vi "RTEH Error Processor.vi"(4 "Valid Default":bool, 6 "Default Action":T2, 8 "Error to Check":errorcluster, 9 "Detect Any Warnings":bool, 10 "Iteration":i32, 11 "Error Handling Info":T2[](array[typedef])) -> (0 "error out":errorcluster, 1 "Loop?":bool, 2 "Classification":string, 5 "Internal Status":cluster{"Status":T1, "Error Code":i32})   [LabVIEW 2024]
doc: "This SubVI exists so that changes made to the underlying error handling code will propagate to existing instances of the Express VI."
uses:
  Controls/RTEH/RTEH Error Options.ctl
  Controls/RTEH/RTEH Shared Error Options.ctl
  Controls/RTEH/RTEH Status Type.ctl
  Controls/Shared/SEH Error Notification Command.ctl
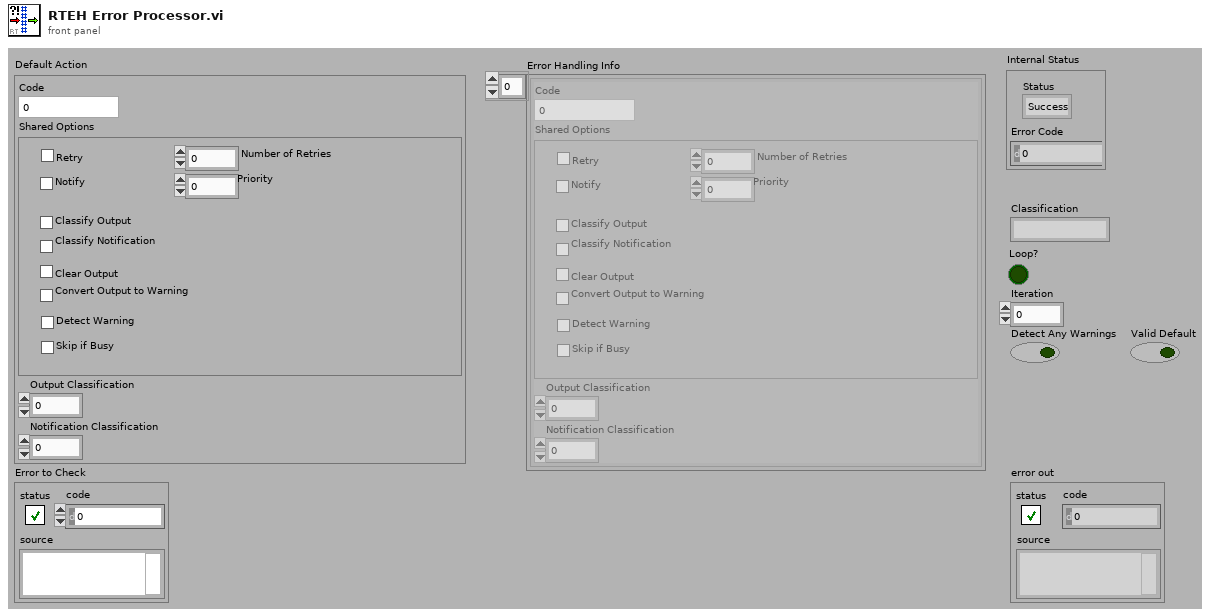
[diagram p1: front panel]
types:
  T1 = typedef "RTEH Status Type.ctl" = enum16{"Success", "Error", "Warning", "Skipped Notification"}
  T2 = typedef "RTEH Error Options.ctl" = cluster{"Code":i32, "Shared Options":T3, "Output Classification":u32, "Notification Classification":u32}
  T3 = typedef "RTEH Shared Error Options.ctl" = cluster{"Number of Retries":i32, "Retry":bool, "Classify Output":bool, "Classify Notification":bool, "Convert Output to Warning":bool, "Clear Output":bool, "Notify":bool, "Priority":i32, "Detect Warning":bool, "Skip if Busy":bool}
  T4 = typedef "SEH Error Notification Command.ctl" = enum16{"Init", "Send Error", "Check Error", "Invalid Command"}
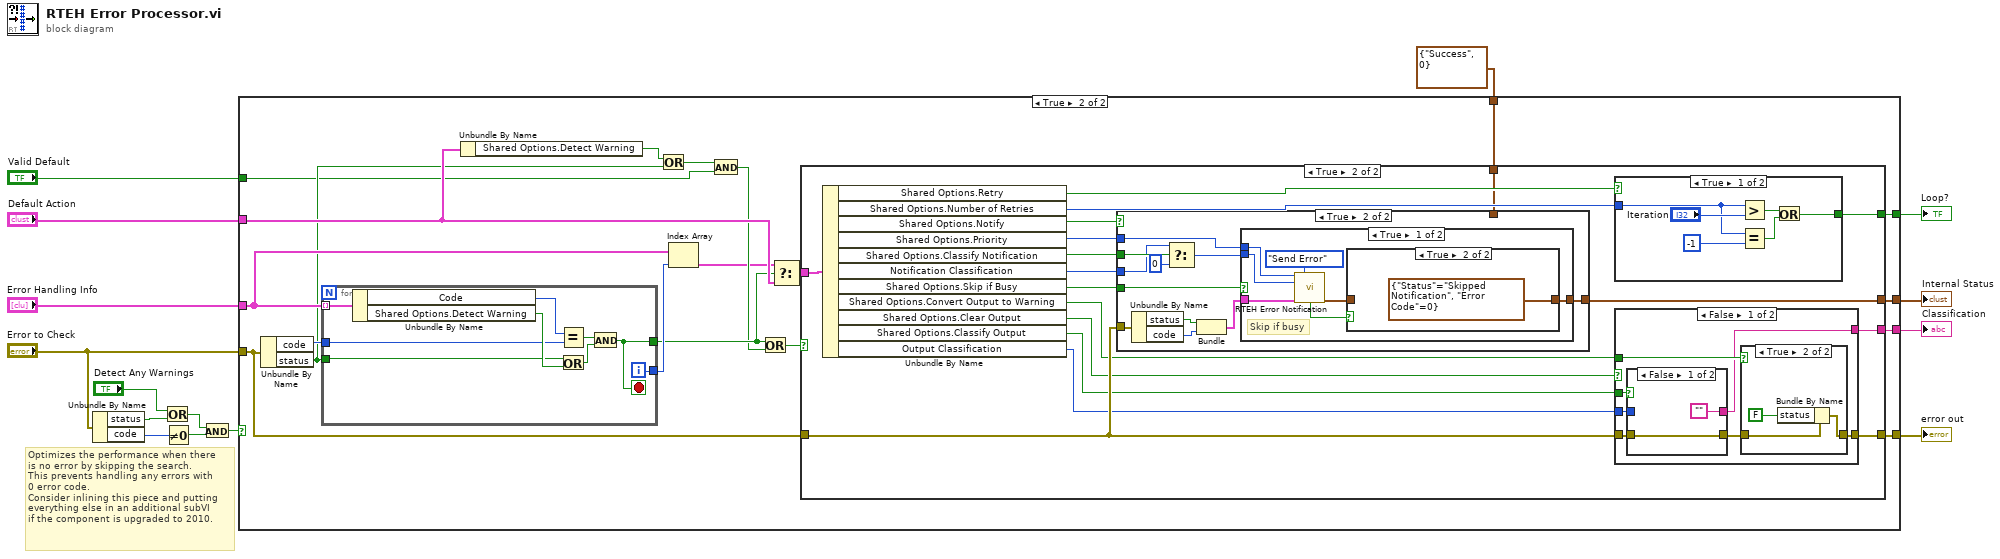
[diagram p0: block diagram]
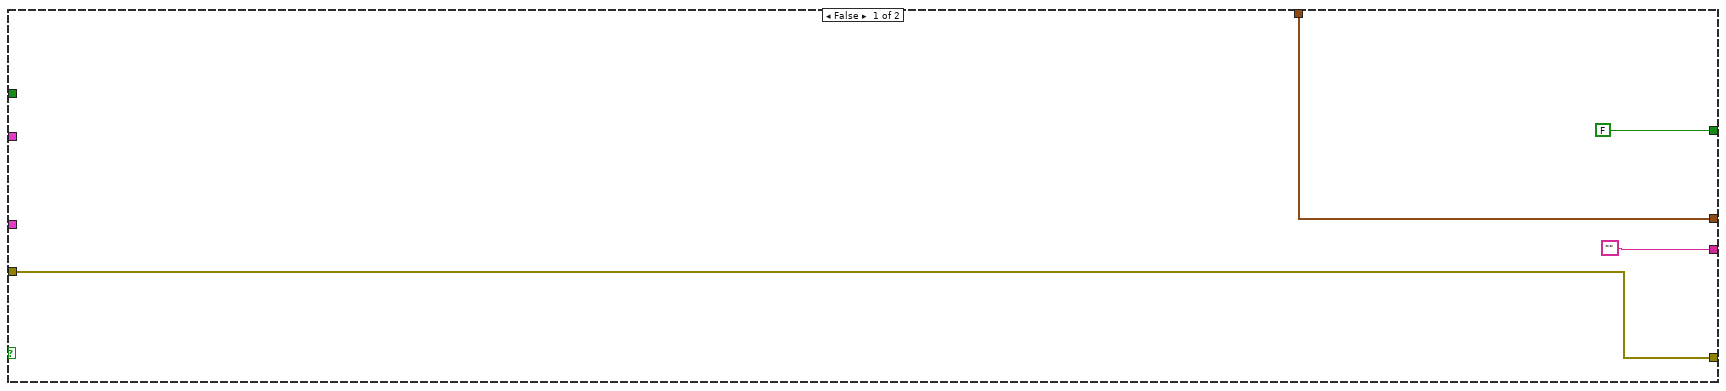
[diagram p2: hidden frame]
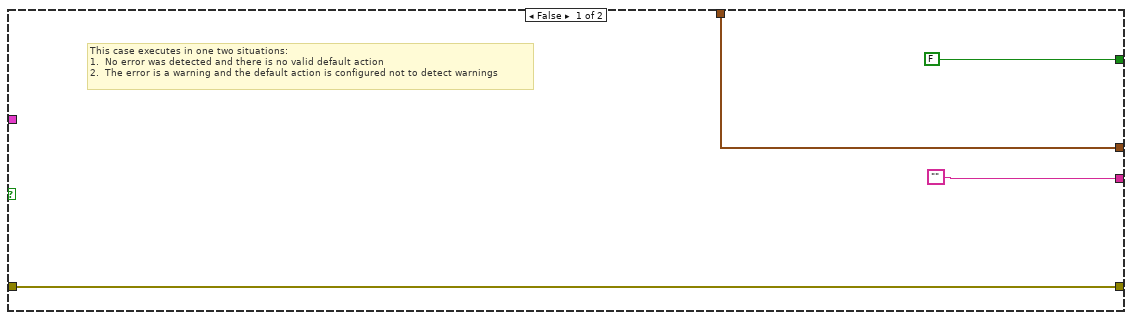
[diagram p3: hidden frame]
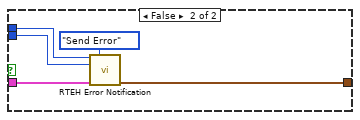
[diagram p6: hidden frame]
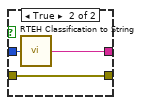
[diagram p8: hidden frame]
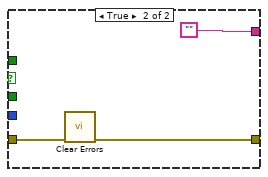
[diagram p9: hidden frame]
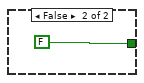
[diagram p10: hidden frame]
diagram:
  # "Optimizes the performance when there\nis no error by skipping the search.\nThis prevents handling any errors with\n0 error code.\nConsider inlining this piece and putting \neverything else in an additional subVI \nif the component is upgraded to 2010."
  n1 = Unbundle By Name("Error to Check") -> ("status"=w8:bool, "code"=w11:i32)
  n2 = Or(x="Detect Any Warnings", y=w8) -> (x .or. y?=w7:bool)
  n3 = Not Equal To 0?(x=w11) -> (x != 0?=w10:bool)
  n4 = And(x=w7, y=w10) -> (x .and. y?=w9:bool)
  n5 = case shown="True" w9 {
    tunnel: "Error Handling Info" -> [_ w38]
    tunnel: "Error to Check" -> [w19 w34]
    tunnel: [w19 w37] -> w14
    tunnel: [FALSE ("T button?") w36] -> w13
    tunnel: "Default Action" -> [_ w31]
    tunnel: "Valid Default" -> [_ w27]
    tunnel: ["" w23] -> w3
    tunnel: [w17 w22] -> w2
    tunnel: cluster{"Status":T1, "Error Code":i32} {"Status"=enum."Success", "Error Code"=0} ("Internal Status") -> [w17 w21]
    frame False {
    }
    frame True {
      n6 = Unbundle By Name(w34) -> ("code"=w33:i32, "status"=w29:bool)
      n7 = for {
        tunnel: w38 -> [w47] mode=indexing
        tunnel: [w43] -> w26
        tunnel: [w45] -> w35
        tunnel: w33 -> [w40]
        tunnel: w29 -> [w39]
        i -> [w45]
        stop <- w43 stop-if-true
        n8 = Unbundle By Name(w47) -> ("Code"=w44:i32, "Shared Options.Detect Warning"=w41:bool)
        n9 = Equal?(x=w44, y=w40) -> (x = y?=w46:bool)
        n10 = Or(x=w39, y=w41) -> (x .or. y?=w42:bool)
        n11 = And(x=w46, y=w42) -> (x .and. y?=w43:bool)
      }
      n12 = Unbundle By Name(w31) -> ("Shared Options.Detect Warning"=w30:bool)
      n13 = Or(x=w30, y=w29) -> (x .or. y?=w28:bool)
      n14 = Index Array(array=w38, index=w35) -> (element=w20:T2)
      n15 = And(x=w28, y=w27) -> (x .and. y?=w25:bool)
      n16 = Or(x=w26, y=w25) -> (x .or. y?=w24:bool)
      n17 = Select(t=w20, s=w26, f=w31) -> (s? t:f=w32:T2)
      n18 = case shown="True" w24 {
        tunnel: [FALSE ("T button?") w69] -> w36
        tunnel: w34 -> [w50 w60]
        tunnel: [w50 w68] -> w37
        tunnel: w32 -> [_ w65]
        tunnel: ["" w55] -> w23
        tunnel: [w49 w54] -> w22
        tunnel: w21 -> [w49 w53]
        frame False {
          # "This case executes in one two situations:\n1.  No error was detected and there is no valid default action\n2.  The error is a warning and the default action is configured not to detect warnings"
        }
        frame True {
          n19 = Unbundle By Name(w65) -> ("Shared Options.Retry"=w67:bool, "Shared Options.Number of Retries"=w66:i32, "Shared Options.Notify"=w64:bool, "Shared Options.Priority"=w63:i32, "Shared Options.Classify Notification"=w62:bool, "Notification Classification"=w61:u32, "Shared Options.Skip if Busy"=w52:bool, "Shared Options.Convert Output to Warning"=w56:bool, "Shared Options.Clear Output"=w59:bool, "Shared Options.Classify Output"=w58:bool, "Output Classification"=w57:u32)
          n20 = case shown="True" w64 {
            tunnel: w63 -> [_ w81]
            tunnel: w60 -> [_ w75]
            tunnel: w62 -> [_ w79]
            tunnel: w61 -> [_ w78]
            tunnel: [w70 w80] -> w54
            tunnel: w53 -> [w70 _]
            tunnel: w52 -> [_ w71]
            frame False {
            }
            frame True {
              n21 = Unbundle By Name(w75) -> ("status"=w74:bool, "code"=w73:i32)
              n22 = Select(t=w78, s=w79, f=u32 0) -> (s? t:f=w76:u32)
              n23 = Bundle("status"=w74, "code"=w73) -> (w72:cluster{"status":bool, "code":i32})  [unwired: 1 in]
              n24 = case shown="True" w71 {
                tunnel: w81 -> [w87 w94]
                tunnel: [w82 w93] -> w80
                tunnel: w76 -> [w86 w92]
                tunnel: w72 -> [w85 w91]
                frame True {
                  # "Skip if busy"
                  n25 = call "RTEH Error Notification.vi"("Priority"=w87, "Command"=SEH_Error_Notification_Command."Send Error", "Classification"=w86, "Error to Send"=w85) -> ("Skipped?"=w84:bool, "Internal Status"=w83:cluster{"Status":T1, "Error Code":i32})  [unwired: 4 in, 6 out]
                  n26 = case shown="True" w84 {
                    tunnel: w83 -> [w89 _]
                    tunnel: [w89 cluster{"Status":T1, "Error Code":i32} {"Status"=enum."Skipped Notification", "Error Code"=0} ("Internal Status")] -> w82
                    frame False {
                    }
                    frame True {
                    }
                  }
                }
                frame False {
                  n27 = call "RTEH Error Notification.vi"("Priority"=w94, "Command"=SEH_Error_Notification_Command."Send Error", "Classification"=w92, "Error to Send"=w91) -> ("Internal Status"=w93:cluster{"Status":T1, "Error Code":i32})  [unwired: 4 in, 7 out]
                }
              }
            }
          }
          n28 = case shown="True" w67 {
            tunnel: [w115 FALSE] -> w69
            tunnel: w66 -> [w116 _]
            frame True {
              n29 = Greater?(x=w116, y="Iteration") -> (0:w120:bool)
              n30 = Equal?(x=w116, y=-1) -> (x = y?=w119:bool)
              n31 = Or(x=w120, y=w119) -> (x .or. y?=w115:bool)
            }
            frame False {
            }
          }
          n32 = case shown="False" w59 {
            tunnel: w60 -> [w100 w114]
            tunnel: [w98 w113] -> w68
            tunnel: w58 -> [w102 _]
            tunnel: w57 -> [w101 _]
            tunnel: w56 -> [w97 _]
            tunnel: [w96 ""] -> w55
            frame False {
              n33 = case shown="False" w102 {
                tunnel: w101 -> [_ w111]
                tunnel: w100 -> [w108 w109]
                tunnel: [w108 w109] -> w99
                tunnel: ["" w110] -> w96
                frame False {
                }
                frame True {
                  n34 = call "RTEH Classification to String.vi"("Classification as Number"=w111) -> ("Classification as String"=w110:string)  [unwired: 14 in]
                }
              }
              n35 = case shown="True" w97 {
                tunnel: w99 -> [w103 w106]
                tunnel: [w103 w105] -> w98
                frame False {
                }
                frame True {
                  n36 = Bundle By Name(cluster=w106, "status"=FALSE) -> (w105:errorcluster)
                }
              }
            }
            frame True {
              n37 = call <vilib>:"Clear Errors.vi"("error in (no error)"=w114) -> ("error out"=w113:errorcluster)  [unwired: 1 in, 5 out]
            }
          }
        }
      }
    }
  }
  "error out" <- w14
  "Loop?" <- w13
  "Classification" <- w3
  "Internal Status" <- w2
